vi "AddDesignPatterns.vi"(0 "ClassWriterNative":refnum<class "ClassWriterNative.lvclass">, 1 "ClassItemRefIn":refnum<vi>, 2 "DesignPatterns":string[](array[string]), 5 "error in (no error)":errorcluster) -> (14 "ClassWriterNative":refnum<class "ClassWriterNative.lvclass">, 15 "ClassItemRefOut":refnum<vi>, 17 "Cancelled":bool, 19 "error out":errorcluster)   [LabVIEW 2020, in "ClassWriterNative.lvclass"]
uses:
  <resource>/Framework/Providers/Open_GDS/ClassProviders/Provider_LvNativeClass/ClassWriterNative_class/ClassWriterNative.lvclass
  <resource>/Framework/Providers/Open_GDS/ClassProviders/Provider_BaseClassInterface/DesignPatternsData.ctl
  <resource>/Framework/Providers/Open_GDS/ClassProviders/Common/LvClass_class/GDSLvClass_PlugIn.ctl
  <resource>/Framework/Providers/Open_GDS/ClassProviders/Common/LvClass_class/GDSLvClass_PlugInTypes.ctl
  <resource>/Framework/Providers/Open_GDS/ClassProviders/Provider_BaseClassInterface/BaseProvider_SubVIs/BaseProvider_DesignPatternsActions.ctl
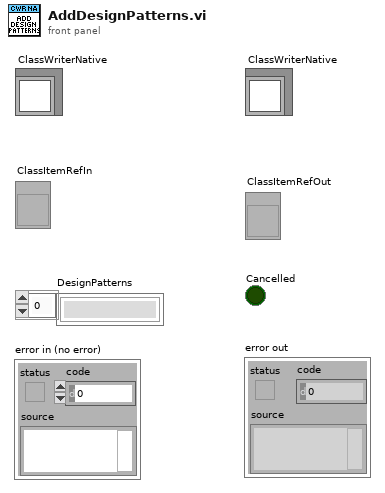
[diagram p1: front panel]
types:
  T1 = typedef "DesignPatternsData.ctl" = cluster{"Type":string, "Patterns":cluster{"ID":string, "Path":path, "Name":string, "Desc":string, "Version":string, "DependenciesID":string[], "OnlyOne":bool}[]}
  T2 = cluster{"Cancel":bool, "ClassProviderName":string, "ClassTemplateUsed":string, "DesignPatterns":T1[], "DataOut":variant, "PlugInVI":path, "DesignPatternID":string, "DesignPatternType":string, "PlugInIDs":string[], "DesignPatternVer":string, "DPIDs":string[], "DpToAdd":cluster{"ID":string, "Path":path, "Name":string, "Desc":string, "Version":string, "DependenciesID":string[], "OnlyOne":bool}[]}
  T3 = cluster{"ID":string, "Path":path, "Name":string, "Desc":string, "Version":string, "DependenciesID":string[], "OnlyOne":bool}[]
  T4 = typedef "GDSLvClass_PlugIn.ctl" = cluster{"Type":T5, "ID":string, "Version":string, "Path":path, "Name":string, "Data":variant}
  T5 = typedef "GDSLvClass_PlugInTypes.ctl" = enum16{"DesignPattern", "MethodTypes"}
  T6 = typedef "BaseProvider_DesignPatternsActions.ctl" = enum16{"AddPatternDialog", "GeneratePattern", "RemovePattern", "CreatePatternMethod", "UpdatePattern"}
  T7 = typedef "GDSLvCLass_ClassSettingsType.ctl" = cluster{"ClassProviderName":string, "ClassTemplateUsed":string, "ClassTemplateVersion":string, "ClassDescription":string, "PlugIns":T4[], "ConnectorPanePattern":string}
  T8 = cluster{"ID":string, "Path":path, "Name":string, "Desc":string, "Version":string, "DependenciesID":string[], "OnlyOne":bool}
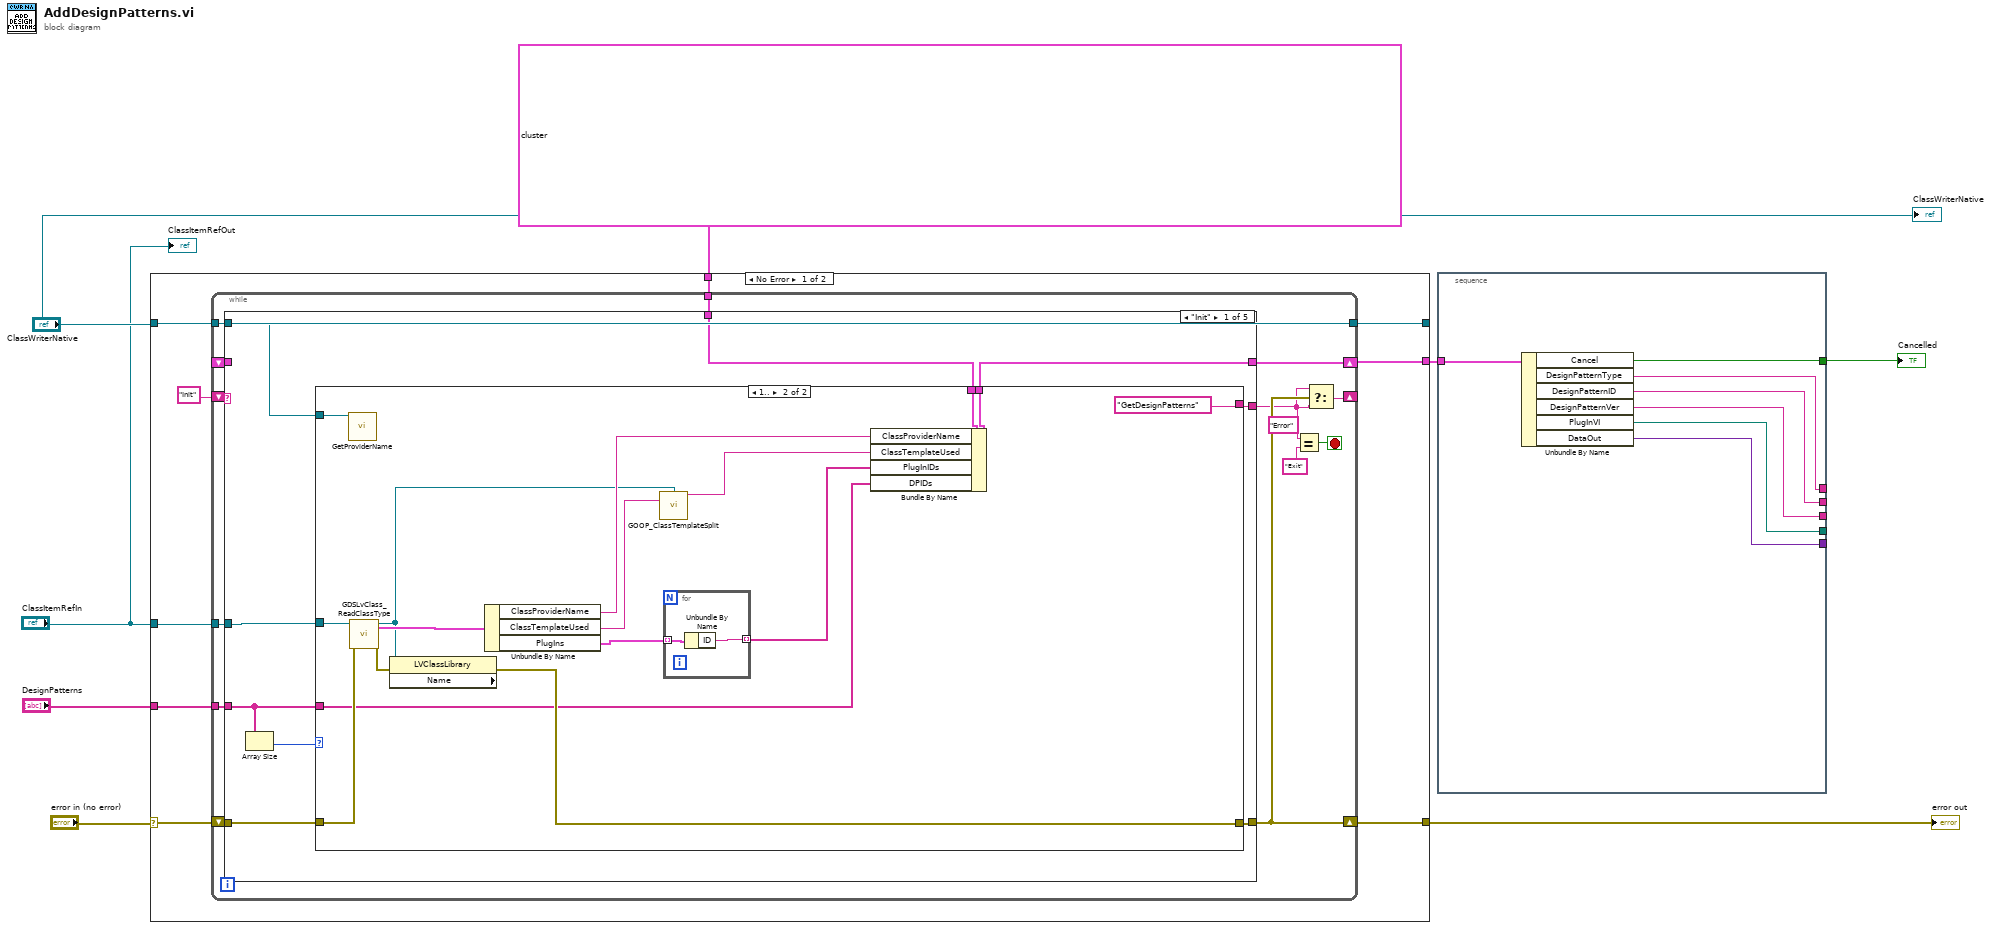
[diagram p0: block diagram]
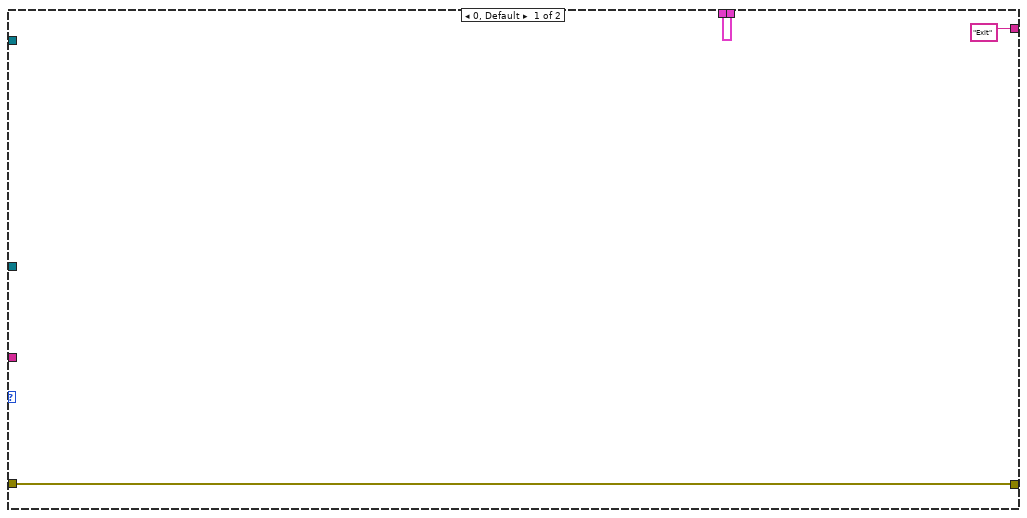
[diagram p2: hidden frame]
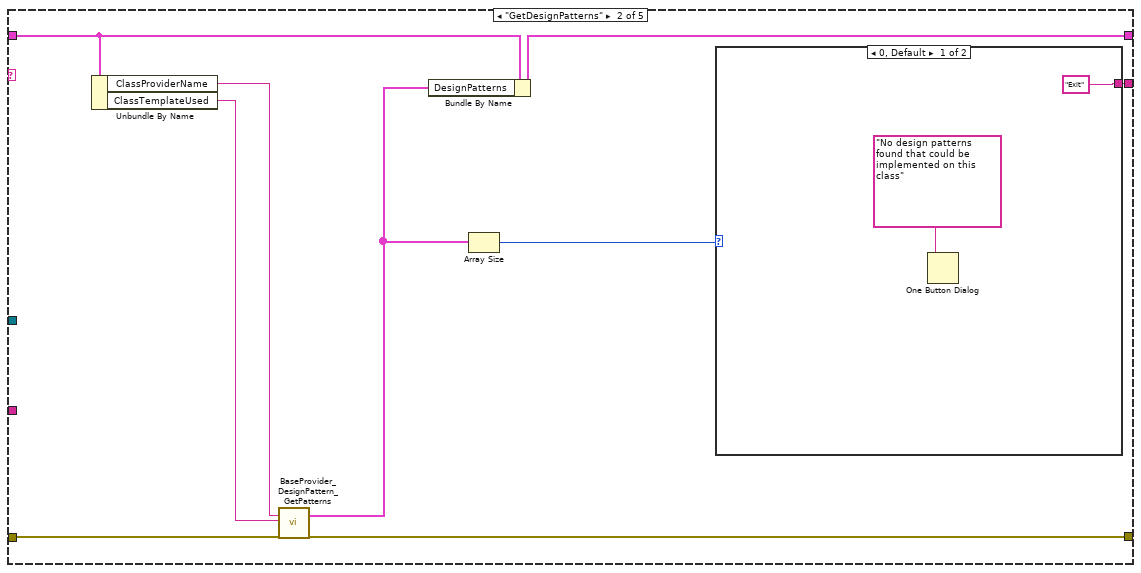
[diagram p3: hidden frame]
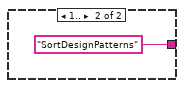
[diagram p4: hidden frame]
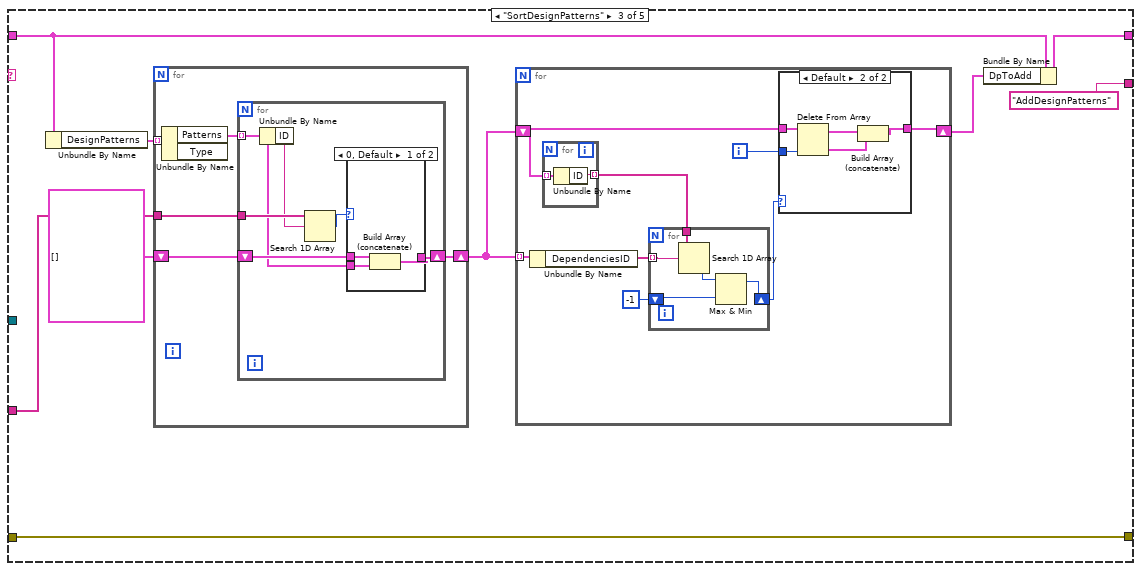
[diagram p5: hidden frame]
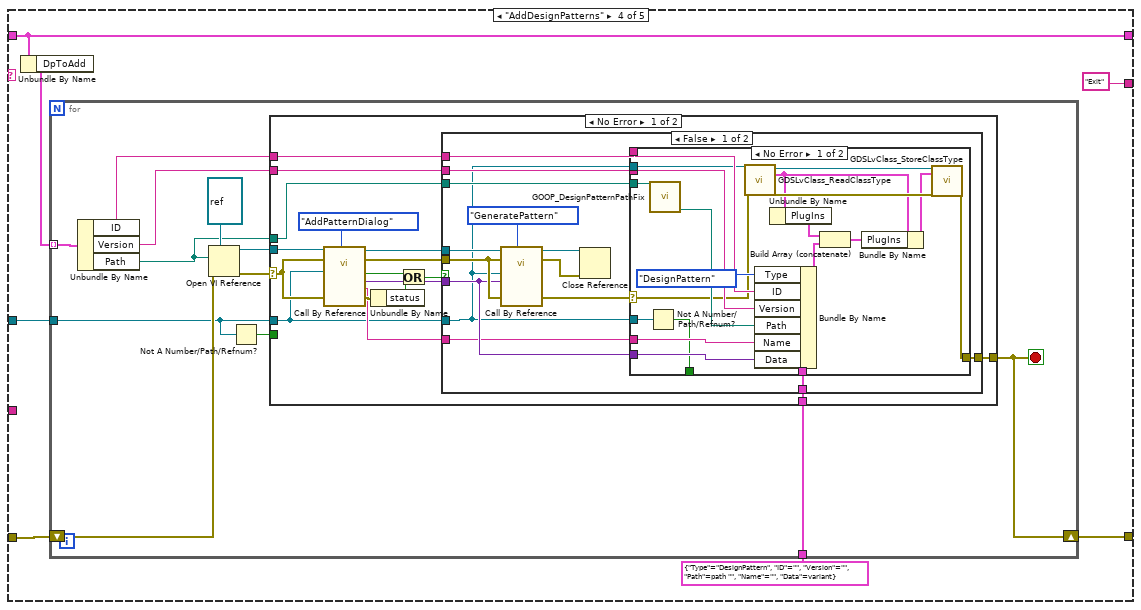
[diagram p8: hidden frame]
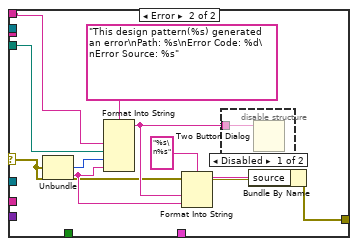
[diagram p9: hidden frame]
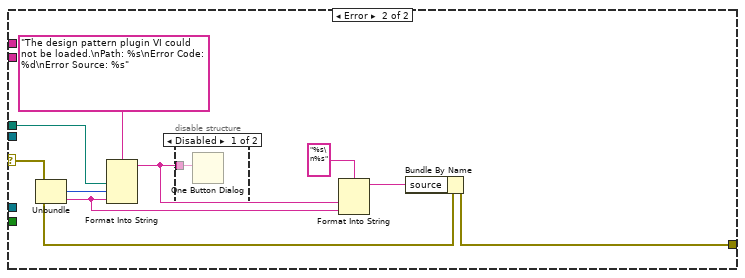
[diagram p12: hidden frame]
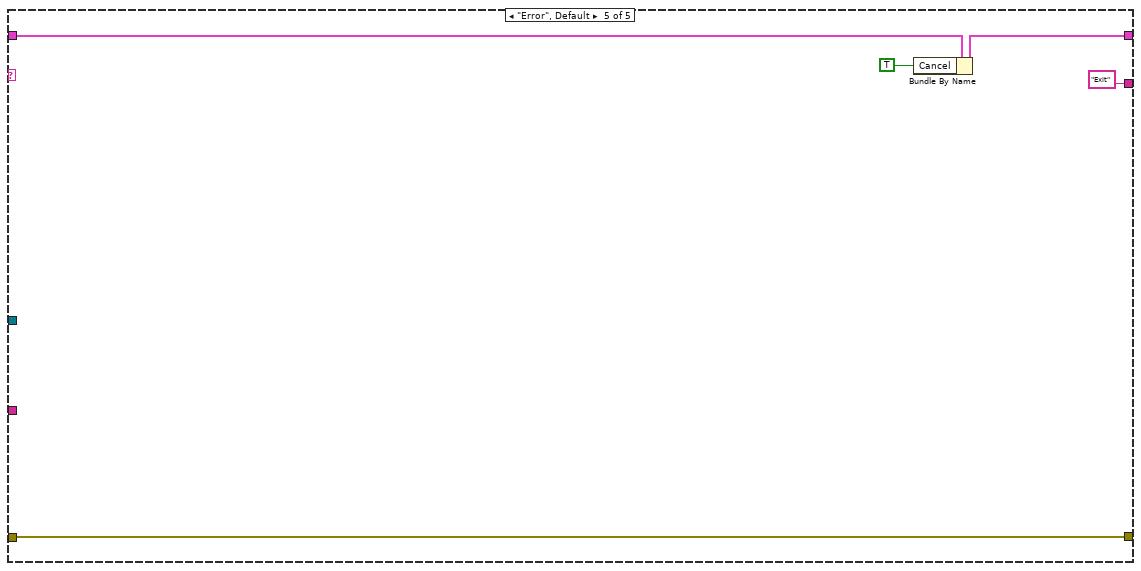
[diagram p14: hidden frame]
diagram:
  n1 = case shown="No Error" "error in (no error)" {
    selector: "error in (no error)" -> [w9 w217]
    tunnel: "ClassWriterNative" -> [w14 w216]
    tunnel: [w17 w217] -> w5
    tunnel: [w15 w216] -> _
    tunnel: T2 {"Cancel"=FALSE, "ClassProviderName"="", "ClassTemplateUsed"="", "DesignPatterns"=[], "DataOut"=variant, "PlugInVI"=path "", "DesignPatternID"="", "DesignPatternType"="", "PlugInIDs"=[], "DesignPatternVer"="", "DPIDs"=[], "DpToAdd"=[]} ("output cluster") -> [w13 _]
    tunnel: "ClassItemRefIn" -> [w12 _]
    tunnel: [w11 _] -> w7
    tunnel: "DesignPatterns" -> [w10 _]
    frame No Error {
      n2 = while {
        shift-right: [w25] -> w17
        shift-left: w9 -> [w31]
        shift-right: [w24] -> _
        shift-left: "Init" -> [w28]
        shift-right: [w29] -> w11
        shift-left: _ -> [w30]
        tunnel: w14 -> [w21]
        tunnel: [w21] -> w15
        tunnel: w13 -> [w20]
        tunnel: w12 -> [w19]
        tunnel: w10 -> [w18]
        stop <- w26 stop-if-true
        n3 = case shown="\"Init\"" w28 {
          tunnel: w30 -> [_ w63 w77 w122 w213]
          tunnel: [w35 w62 w76 w122 w212] -> w29
          tunnel: w31 -> [w38 w68 w80 w124 w214]
          tunnel: [w37 w65 w80 w120 w214] -> w25
          tunnel: w21 -> [w32 _ _ _ _]
          tunnel: [w40 w70 "AddDesignPatterns" "Exit" "Exit"] -> w23
          tunnel: w20 -> [w36 _ _ _ _]
          tunnel: w19 -> [w39 _ _ w123 _]
          tunnel: w18 -> [w34 _ w79 _ _]
          frame "Init" {
            n4 = Array Size(array=w34) -> (size(s)=w33:i32)
            n5 = case shown="1.." w33 {
              tunnel: ["Exit" "GetDesignPatterns"] -> w40
              tunnel: w39 -> [_ w58]
              tunnel: w38 -> [w41 w57]
              tunnel: [w41 w54] -> w37
              tunnel: w36 -> [w43 w52]
              tunnel: [w43 w51] -> w35
              tunnel: w34 -> [_ w48]
              tunnel: w32 -> [_ w47]
              frame 0, Default {
              }
              frame 1.. {
                n6 = call-dynamic "GetProviderName.vi"("ClassWriterNative in"=w47) -> ()  [unwired: 16 in, 3 out]
                n7 = call <resource>:"GDSLvClass_ReadClassType.vi"("Class Refnum In"=w58, "error in (no error)"=w57) -> ("Class Refnum Out"=w44:refnum<vi>, "ClassSettings"=w56:T7, "error out"=w55:errorcluster)  [unwired: 15 in]
                n8 = property class="LVClassLibrary" props=["Name"](reference=w44, error in=w55) -> (error out=w54:errorcluster)  [unwired: 2 out]
                n9 = Unbundle By Name(w56) -> ("ClassProviderName"=w53:string, "ClassTemplateUsed"=w46:string, "PlugIns"=w50:T4[])
                n10 = call <resource>:"GOOP_ClassTemplateSplit.vi"("ClassItemRefIn"=w44, "FullClassTemplate"=w46) -> ("StandardTemplate"=w45:string)  [unwired: 12 in, 1 out]
                n11 = for {
                  tunnel: w50 -> [w61] mode=indexing
                  tunnel: [w60] -> w49 mode=indexing
                  n12 = Unbundle By Name(w61) -> ("ID"=w60:string)
                }
                n13 = Bundle By Name(cluster=w52, "ClassProviderName"=w53, "ClassTemplateUsed"=w45, "PlugInIDs"=w49, "DPIDs"=w48) -> (w51:T2)
              }
            }
          }
          frame "GetDesignPatterns" {
            n14 = Unbundle By Name(w63) -> ("ClassProviderName"=w67:string, "ClassTemplateUsed"=w66:string)
            n15 = call <resource>:"BaseProvider_DesignPattern_GetPatterns.vi"("FilterOnProviders(Ignored If Empty)"=w67, "FilterOnTemplate(Ignored If Empty)"=w66, "error in (no error)"=w68) -> ("DesignPatterns"=w64:T1[], "error out"=w65:errorcluster)  [unwired: 15 in]
            n16 = Bundle By Name(cluster=w63, "DesignPatterns"=w64) -> (w62:T2)
            n17 = Array Size(array=w64) -> (size(s)=w69:i32)
            n18 = case shown="0, Default" w69 {
              tunnel: ["Exit" "SortDesignPatterns"] -> w70
              frame 0, Default {
                n19 = One Button Dialog(message="No design patterns found that could be implemented on this class" ("format string")) -> ()  [unwired: 1 in, 1 out]
              }
              frame 1.. {
              }
            }
          }
          frame "SortDesignPatterns" {
            n20 = Unbundle By Name(w77) -> ("DesignPatterns"=w81:T1[])
            n21 = for {
              tunnel: w81 -> [w108] mode=indexing
              tunnel: w79 -> [w106]
              shift-right: [w104] -> w78
              shift-left: T3 [] -> [w105]
              n22 = Unbundle By Name(w108) -> ("Patterns"=w107:T3)  [unwired: 1 out]
              n23 = for {
                tunnel: w107 -> [w109] mode=indexing
                tunnel: w106 -> [w114]
                shift-right: [w110] -> w104
                shift-left: w105 -> [w111]
                n24 = Unbundle By Name(w109) -> ("ID"=w113:string)
                n25 = Search 1D Array(1D array=w114, element=w113) -> (index of element=w112:i32)  [unwired: 1 in]
                n26 = case shown="0, Default" w112 {
                  tunnel: w111 -> [w117 w118]
                  tunnel: [w116 w118] -> w110
                  tunnel: w109 -> [w115 _]
                  frame 0, Default {
                    n27 = Build Array (concatenate)(w117, w115) -> (w116:T3)
                  }
                  frame -1 {
                  }
                }
              }
            }
            n28 = for {
              tunnel: w78 -> [w90] mode=indexing
              shift-right: [w84] -> w75
              shift-left: w78 -> [w86]
              i -> [w83]
              n29 = Unbundle By Name(w90) -> ("DependenciesID"=w89:string[])
              n30 = for {
                tunnel: w86 -> [w103] mode=indexing
                tunnel: [w102] -> w88 mode=indexing
                n31 = Unbundle By Name(w103) -> ("ID"=w102:string)
              }
              n32 = for {
                tunnel: w89 -> [w101] mode=indexing
                tunnel: w88 -> [w100]
                shift-right: [w97] -> w85
                shift-left: -1 -> [w98]
                n33 = Search 1D Array(1D array=w100, element=w101) -> (index of element=w99:i32)  [unwired: 1 in]
                n34 = Max & Min(x=w99, y=w98) -> (max(x,y)=w97:i32)  [unwired: 1 out]
              }
              n35 = case shown="Default" w85 {
                tunnel: w86 -> [w91 w96]
                tunnel: [w91 w92] -> w84
                tunnel: w83 -> [_ w95]
                frame -1 {
                }
                frame Default {
                  n36 = Delete From Array(array=w96, index=w95) -> (deleted portion=w93:T8, array with subset deleted=w94:T3)  [unwired: 1 in]
                  n37 = Build Array (concatenate)(w94, w93) -> (w92:T3)
                }
              }
            }
            n38 = Bundle By Name(cluster=w77, "DpToAdd"=w75) -> (w76:T2)
          }
          frame "AddDesignPatterns" {
            n39 = Unbundle By Name(w122) -> ("DpToAdd"=w125:T3)
            n40 = for {
              tunnel: w125 -> [w133] mode=indexing
              shift-right: [w126] -> w120
              shift-left: w124 -> [w132]
              tunnel: w123 -> [w128]
              tunnel: T4 {"Type"=enum."DesignPattern", "ID"="", "Version"="", "Path"=path "", "Name"="", "Data"=variant} ("PlugIn") -> [w131]
              stop <- w126 stop-if-true
              n41 = Unbundle By Name(w133) -> ("ID"=w130:string, "Version"=w129:string, "Path"=w134:path)
              n42 = Open VI Reference(type specifier VI Refnum (for type only)=refnum<vi> refnum, vi path=w134, error in (no error)=w132) -> (vi reference=w136:refnum<vi>, error out=w135:errorcluster)  [unwired: 3 in]
              n43 = Not A Number/Path/Refnum?(number/path/refnum=w128) -> (NaN/Path/Refnum?=w127:bool)
              n44 = case shown="No Error" w135 {
                selector: w135 -> [w146 w206]
                tunnel: w136 -> [w154 _]
                tunnel: w134 -> [w141 w207]
                tunnel: w128 -> [w139 _]
                tunnel: w131 -> [w144 _]
                tunnel: w130 -> [w143 _]
                tunnel: w129 -> [w142 _]
                tunnel: w127 -> [_ _]
                tunnel: [w138 w201] -> w126
                frame No Error {
                  n45 = call-by-ref "?"(reference=w154, error in=w146, "Action"=BaseProvider_DesignPatternsActions."AddPatternDialog", 8:"error in (no error)"=w146, "ClassRefToActOn"=w139) -> (reference out=w148:refnum<vi>, error out=w147:errorcluster, 0:"error out"=w153:errorcluster, "Name"=w140:string, "DataOut"=w145:variant, "Cancelled"=w152:bool)  [unwired: 5 in]
                  n46 = Unbundle By Name(w153) -> ("status"=w150:bool)
                  n47 = Or(x=w152, y=w150) -> (x .or. y?=w149:bool)
                  n48 = case shown="False" w149 {
                    tunnel: w148 -> [w168 _]
                    tunnel: w139 -> [w156 _]
                    tunnel: w147 -> [w166 w200]
                    tunnel: w145 -> [w161 _]
                    tunnel: w144 -> [w162 _]
                    tunnel: w143 -> [w160 _]
                    tunnel: w142 -> [w159 _]
                    tunnel: w141 -> [w158 _]
                    tunnel: w140 -> [w157 _]
                    tunnel: [w155 w200] -> w138
                    frame False {
                      n49 = call-by-ref "?"(reference=w168, error in=w166, "Action"=BaseProvider_DesignPatternsActions."GeneratePattern", 8:"error in (no error)"=w166, "DataIn"=w161, "ClassRefToActOn"=w156) -> (reference out=w165:refnum<vi>, error out=w164:errorcluster, 0:"error out"=w163:errorcluster)  [unwired: 4 in, 3 out]
                      n50 = Close Reference(reference=w165, error in (no error)=w164) -> ()  [unwired: 1 out]
                      n51 = case shown="No Error" w163 {
                        selector: w163 -> [w169 w190]
                        tunnel: w162 -> [w180 _]
                        tunnel: w161 -> [w179 _]
                        tunnel: w160 -> [w178 w196]
                        tunnel: w159 -> [w177 _]
                        tunnel: w158 -> [w172 w195]
                        tunnel: w156 -> [w176 _]
                        tunnel: w157 -> [w175 _]
                        tunnel: w156 -> [w174 _]
                        tunnel: [w173 _] -> _
                        tunnel: [w170 w189] -> w155
                        frame No Error {
                          n52 = Not A Number/Path/Refnum?(number/path/refnum=w174) -> (NaN/Path/Refnum?=w173:bool)
                          n53 = call <resource>:"GOOP_DesignPatternPathFix.vi"("ViPathIn"=w172) -> ("RelativeVIPathOut(ToStoreInLvClass)"=w171:path)  [unwired: 6 in, 4 out]
                          n54 = call <resource>:"GDSLvClass_ReadClassType.vi"("Class Refnum In"=w176, "error in (no error)"=w169) -> ("Class Refnum Out"=w188:refnum<vi>, "ClassSettings"=w185:T7, "error out"=w187:errorcluster)  [unwired: 15 in]
                          n55 = Bundle By Name(cluster=w180, "Type"=GDSLvClass_PlugInTypes."DesignPattern", "ID"=w178, "Version"=w177, "Path"=w171, "Name"=w175, "Data"=w179) -> (w182:T4)
                          n56 = Unbundle By Name(w185) -> ("PlugIns"=w184:T4[])
                          n57 = Build Array (concatenate)(w184, w182) -> (w183:T4[])
                          n58 = Bundle By Name(cluster=w185, "PlugIns"=w183) -> (w186:T7)
                          n59 = call <resource>:"GDSLvClass_StoreClassType.vi"("Class Refnum In"=w188, "ClassSettings"=w186, "error in (no error)"=w187) -> ("error out"=w170:errorcluster)  [unwired: 15 in, 1 out]
                        }
                        frame Error {
                          n60 = Unbundle(w190) -> ("code"=w197:i32, "source"=w191:string)  [unwired: 1 out]
                          n61 = Format Into String(format string="This design pattern(%s) generated an error\nPath: %s\nError Code: %d\nError Source: %s" ("message"), w196, w195, w197, w191) -> (resulting string=w192:string)  [unwired: 2 in, 1 out]
                          n62 = Format Into String(format string="%s\n%s", w192, w191) -> (resulting string=w193:string)  [unwired: 2 in, 1 out]
                          n63 = disable-structure shown="Disabled" {
                            disable-tunnel: w192 -> [w199 _]
                            frame Disabled {
                              n64 = Two Button Dialog(message=w199) -> ()  [unwired: 2 in, 1 out]
                            }
                            frame Enabled {
                            }
                          }
                          n65 = Bundle By Name(cluster=w190, "source"=w193) -> (w189:errorcluster)
                        }
                      }
                    }
                    frame True {
                    }
                  }
                }
                frame Error {
                  n66 = Unbundle(w206) -> ("code"=w208:i32, "source"=w203:string)  [unwired: 1 out]
                  n67 = Format Into String(format string="The design pattern plugin VI could not be loaded.\nPath: %s\nError Code: %d\nError Source: %s" ("message"), w207, w208, w203) -> (resulting string=w204:string)  [unwired: 2 in, 1 out]
                  n68 = disable-structure shown="Disabled" {
                    disable-tunnel: w204 -> [w210 _]
                    frame Disabled {
                      n69 = One Button Dialog(message=w210) -> ()  [unwired: 1 in, 1 out]
                    }
                    frame Enabled {
                    }
                  }
                  n70 = Format Into String(format string="%s\n%s", w204, w203) -> (resulting string=w202:string)  [unwired: 2 in, 1 out]
                  n71 = Bundle By Name(cluster=w206, "source"=w202) -> (w201:errorcluster)
                }
              }
            }
          }
          frame "Error", Default {
            n72 = Bundle By Name(cluster=w213, "Cancel"=TRUE) -> (w212:T2)
          }
        }
        n73 = Equal?(x=w23, y="Exit") -> (x = y?=w26:bool)
        n74 = Select(t="Error", s=w25, f=w23) -> (s? t:f=w24:string)
      }
    }
    frame Error {
    }
  }
  "error out" <- w5
  n75 = stacked-sequence {
    tunnel: w7 -> [w224]
    tunnel: [w223] -> w6
    tunnel: [w222] -> _
    tunnel: [w221] -> _
    tunnel: [w220] -> _
    tunnel: [w219] -> _
    tunnel: [w218] -> _
    frame #0 {
      n76 = Unbundle By Name(w224) -> ("Cancel"=w223:bool, "DesignPatternType"=w219:string, "DesignPatternID"=w220:string, "DesignPatternVer"=w218:string, "PlugInVI"=w222:path, "DataOut"=w221:variant)
    }
  }
  "Cancelled" <- w6
  "ClassWriterNative" <- "ClassWriterNative"
  "ClassItemRefOut" <- "ClassItemRefIn"
